vi "Change Camera Configuration.vi"(8 "error in (no error)":errorcluster, 10 "Camera Controls":T1={"VideoMode"=81, "Brightness"=150, "Sharpness"=50, "White Balance"=8000, "Saturation"=75, "Exposure"=5} {"VideoMode" items=["640 x 480 YUY 2 30.00 fps", "640 x 480 YUY 2 20.00 fps", "640 x 480 YUY 2 15.00 fps", "640 x 480 YUY 2 10.00 fps", "640 x 480 YUY 2 7.50 fps", "1280 x 720 YUY 2 10.00 fps", "1280 x 720 YUY 2 7.50 fps", "960 x 544 YUY 2 15.00 fps", "960 x 544 YUY 2 10.00 fps", "960 x 544 YUY 2 7.50 fps", "800 x 448 YUY 2 20.00 fps", "800 x 448 YUY 2 15.00 fps", "800 x 448 YUY 2 10.00 fps", "800 x 448 YUY 2 7.50 fps", "640 x 360 YUY 2 30.00 fps", "640 x 360 YUY 2 20.00 fps", "640 x 360 YUY 2 15.00 fps", "640 x 360 YUY 2 10.00 fps", "640 x 360 YUY 2 7.50 fps", "424 x 240 YUY 2 30.00 fps", "424 x 240 YUY 2 20.00 fps", "424 x 240 YUY 2 15.00 fps", "424 x 240 YUY 2 10.00 fps", "424 x 240 YUY 2 7.50 fps", "352 x 288 YUY 2 30.00 fps", "352 x 288 YUY 2 20.00 fps", "352 x 288 YUY 2 15.00 fps", "352 x 288 YUY 2 10.00 fps", "352 x 288 YUY 2 7.50 fps", "320 x 240 YUY 2 30.00 fps", "320 x 240 YUY 2 20.00 fps", "320 x 240 YUY 2 15.00 fps", "320 x 240 YUY 2 10.00 fps", "320 x 240 YUY 2 7.50 fps", "800 x 600 YUY 2 15.00 fps", "800 x 600 YUY 2 10.00 fps", "800 x 600 YUY 2 7.50 fps", "176 x 144 YUY 2 30.00 fps", "176 x 144 YUY 2 20.00 fps", "176 x 144 YUY 2 15.00 fps", "176 x 144 YUY 2 10.00 fps", "176 x 144 YUY 2 7.50 fps", "160 x 120 YUY 2 30.00 fps", "160 x 120 YUY 2 20.00 fps", "160 x 120 YUY 2 15.00 fps", "160 x 120 YUY 2 10.00 fps", "160 x 120 YUY 2 7.50 fps", "1280 x 800 YUY 2 10.00 fps", "640 x 480 JPEG 30.00 fps", "640 x 480 JPEG 20.00 fps", "640 x 480 JPEG 15.00 fps", "640 x 480 JPEG 10.00 fps", "640 x 480 JPEG 7.50 fps", "1280 x 720 JPEG 30.00 fps", "1280 x 720 JPEG 20.00 fps", "1280 x 720 JPEG 15.00 fps", "1280 x 720 JPEG 10.00 fps", "1280 x 720 JPEG 7.50 fps", "960 x 544 JPEG 30.00 fps", "960 x 544 JPEG 20.00 fps", "960 x 544 JPEG 15.00 fps", "960 x 544 JPEG 10.00 fps", "960 x 544 JPEG 7.50 fps", "800 x 448 JPEG 30.00 fps", "800 x 448 JPEG 20.00 fps", "800 x 448 JPEG 15.00 fps", "800 x 448 JPEG 10.00 fps", "800 x 448 JPEG 7.50 fps", "640 x 360 JPEG 30.00 fps", "640 x 360 JPEG 20.00 fps", "640 x 360 JPEG 15.00 fps", "640 x 360 JPEG 10.00 fps", "640 x 360 JPEG 7.50 fps", "800 x 600 JPEG 30.00 fps", "800 x 600 JPEG 20.00 fps", "800 x 600 JPEG 15.00 fps", "800 x 600 JPEG 10.00 fps", "800 x 600 JPEG 7.50 fps", "416 x 240 JPEG 30.00 fps", "416 x 240 JPEG 20.00 fps", "416 x 240 JPEG 15.00 fps", "416 x 240 JPEG 10.00 fps", "416 x 240 JPEG 7.50 fps", "352 x 288 JPEG 30.00 fps", "352 x 288 JPEG 20.00 fps", "352 x 288 JPEG 15.00 fps", "352 x 288 JPEG 10.00 fps", "352 x 288 JPEG 7.50 fps", "176 x 144 JPEG 30.00 fps", "176 x 144 JPEG 20.00 fps", "176 x 144 JPEG 15.00 fps", "176 x 144 JPEG 10.00 fps", "176 x 144 JPEG 7.50 fps", "320 x 240 JPEG 30.00 fps", "320 x 240 JPEG 20.00 fps", "320 x 240 JPEG 15.00 fps", "320 x 240 JPEG 10.00 fps", "320 x 240 JPEG 7.50 fps", "160 x 120 JPEG 30.00 fps", "160 x 120 JPEG 20.00 fps", "160 x 120 JPEG 15.00 fps", "160 x 120 JPEG 10.00 fps", "160 x 120 JPEG 7.50 fps"]}, 11 "Refnum In":T3={"Session"="", "Camera Settings"={"VideoMode"=81, "Brightness"=0, "Sharpness"=0, "White Balance"=0, "Saturation"=0, "Exposure"=0}} {"Camera Settings"."VideoMode" items=["640 x 480 YUY 2 30.00 fps", "640 x 480 YUY 2 20.00 fps", "640 x 480 YUY 2 15.00 fps", "640 x 480 YUY 2 10.00 fps", "640 x 480 YUY 2 7.50 fps", "1280 x 720 YUY 2 10.00 fps", "1280 x 720 YUY 2 7.50 fps", "960 x 544 YUY 2 15.00 fps", "960 x 544 YUY 2 10.00 fps", "960 x 544 YUY 2 7.50 fps", "800 x 448 YUY 2 20.00 fps", "800 x 448 YUY 2 15.00 fps", "800 x 448 YUY 2 10.00 fps", "800 x 448 YUY 2 7.50 fps", "640 x 360 YUY 2 30.00 fps", "640 x 360 YUY 2 20.00 fps", "640 x 360 YUY 2 15.00 fps", "640 x 360 YUY 2 10.00 fps", "640 x 360 YUY 2 7.50 fps", "424 x 240 YUY 2 30.00 fps", "424 x 240 YUY 2 20.00 fps", "424 x 240 YUY 2 15.00 fps", "424 x 240 YUY 2 10.00 fps", "424 x 240 YUY 2 7.50 fps", "352 x 288 YUY 2 30.00 fps", "352 x 288 YUY 2 20.00 fps", "352 x 288 YUY 2 15.00 fps", "352 x 288 YUY 2 10.00 fps", "352 x 288 YUY 2 7.50 fps", "320 x 240 YUY 2 30.00 fps", "320 x 240 YUY 2 20.00 fps", "320 x 240 YUY 2 15.00 fps", "320 x 240 YUY 2 10.00 fps", "320 x 240 YUY 2 7.50 fps", "800 x 600 YUY 2 15.00 fps", "800 x 600 YUY 2 10.00 fps", "800 x 600 YUY 2 7.50 fps", "176 x 144 YUY 2 30.00 fps", "176 x 144 YUY 2 20.00 fps", "176 x 144 YUY 2 15.00 fps", "176 x 144 YUY 2 10.00 fps", "176 x 144 YUY 2 7.50 fps", "160 x 120 YUY 2 30.00 fps", "160 x 120 YUY 2 20.00 fps", "160 x 120 YUY 2 15.00 fps", "160 x 120 YUY 2 10.00 fps", "160 x 120 YUY 2 7.50 fps", "1280 x 800 YUY 2 10.00 fps", "640 x 480 JPEG 30.00 fps", "640 x 480 JPEG 20.00 fps", "640 x 480 JPEG 15.00 fps", "640 x 480 JPEG 10.00 fps", "640 x 480 JPEG 7.50 fps", "1280 x 720 JPEG 30.00 fps", "1280 x 720 JPEG 20.00 fps", "1280 x 720 JPEG 15.00 fps", "1280 x 720 JPEG 10.00 fps", "1280 x 720 JPEG 7.50 fps", "960 x 544 JPEG 30.00 fps", "960 x 544 JPEG 20.00 fps", "960 x 544 JPEG 15.00 fps", "960 x 544 JPEG 10.00 fps", "960 x 544 JPEG 7.50 fps", "800 x 448 JPEG 30.00 fps", "800 x 448 JPEG 20.00 fps", "800 x 448 JPEG 15.00 fps", "800 x 448 JPEG 10.00 fps", "800 x 448 JPEG 7.50 fps", "640 x 360 JPEG 30.00 fps", "640 x 360 JPEG 20.00 fps", "640 x 360 JPEG 15.00 fps", "640 x 360 JPEG 10.00 fps", "640 x 360 JPEG 7.50 fps", "800 x 600 JPEG 30.00 fps", "800 x 600 JPEG 20.00 fps", "800 x 600 JPEG 15.00 fps", "800 x 600 JPEG 10.00 fps", "800 x 600 JPEG 7.50 fps", "416 x 240 JPEG 30.00 fps", "416 x 240 JPEG 20.00 fps", "416 x 240 JPEG 15.00 fps", "416 x 240 JPEG 10.00 fps", "416 x 240 JPEG 7.50 fps", "352 x 288 JPEG 30.00 fps", "352 x 288 JPEG 20.00 fps", "352 x 288 JPEG 15.00 fps", "352 x 288 JPEG 10.00 fps", "352 x 288 JPEG 7.50 fps", "176 x 144 JPEG 30.00 fps", "176 x 144 JPEG 20.00 fps", "176 x 144 JPEG 15.00 fps", "176 x 144 JPEG 10.00 fps", "176 x 144 JPEG 7.50 fps", "320 x 240 JPEG 30.00 fps", "320 x 240 JPEG 20.00 fps", "320 x 240 JPEG 15.00 fps", "320 x 240 JPEG 10.00 fps", "320 x 240 JPEG 7.50 fps", "160 x 120 JPEG 30.00 fps", "160 x 120 JPEG 20.00 fps", "160 x 120 JPEG 15.00 fps", "160 x 120 JPEG 10.00 fps", "160 x 120 JPEG 7.50 fps"]}) -> (0 "error out":errorcluster, 2 "Camera Controls Out":T1={"VideoMode"=81, "Brightness"=150, "Sharpness"=50, "White Balance"=8000, "Saturation"=75, "Exposure"=5} {"VideoMode" items=["640 x 480 YUY 2 30.00 fps", "640 x 480 YUY 2 20.00 fps", "640 x 480 YUY 2 15.00 fps", "640 x 480 YUY 2 10.00 fps", "640 x 480 YUY 2 7.50 fps", "1280 x 720 YUY 2 10.00 fps", "1280 x 720 YUY 2 7.50 fps", "960 x 544 YUY 2 15.00 fps", "960 x 544 YUY 2 10.00 fps", "960 x 544 YUY 2 7.50 fps", "800 x 448 YUY 2 20.00 fps", "800 x 448 YUY 2 15.00 fps", "800 x 448 YUY 2 10.00 fps", "800 x 448 YUY 2 7.50 fps", "640 x 360 YUY 2 30.00 fps", "640 x 360 YUY 2 20.00 fps", "640 x 360 YUY 2 15.00 fps", "640 x 360 YUY 2 10.00 fps", "640 x 360 YUY 2 7.50 fps", "424 x 240 YUY 2 30.00 fps", "424 x 240 YUY 2 20.00 fps", "424 x 240 YUY 2 15.00 fps", "424 x 240 YUY 2 10.00 fps", "424 x 240 YUY 2 7.50 fps", "352 x 288 YUY 2 30.00 fps", "352 x 288 YUY 2 20.00 fps", "352 x 288 YUY 2 15.00 fps", "352 x 288 YUY 2 10.00 fps", "352 x 288 YUY 2 7.50 fps", "320 x 240 YUY 2 30.00 fps", "320 x 240 YUY 2 20.00 fps", "320 x 240 YUY 2 15.00 fps", "320 x 240 YUY 2 10.00 fps", "320 x 240 YUY 2 7.50 fps", "800 x 600 YUY 2 15.00 fps", "800 x 600 YUY 2 10.00 fps", "800 x 600 YUY 2 7.50 fps", "176 x 144 YUY 2 30.00 fps", "176 x 144 YUY 2 20.00 fps", "176 x 144 YUY 2 15.00 fps", "176 x 144 YUY 2 10.00 fps", "176 x 144 YUY 2 7.50 fps", "160 x 120 YUY 2 30.00 fps", "160 x 120 YUY 2 20.00 fps", "160 x 120 YUY 2 15.00 fps", "160 x 120 YUY 2 10.00 fps", "160 x 120 YUY 2 7.50 fps", "1280 x 800 YUY 2 10.00 fps", "640 x 480 JPEG 30.00 fps", "640 x 480 JPEG 20.00 fps", "640 x 480 JPEG 15.00 fps", "640 x 480 JPEG 10.00 fps", "640 x 480 JPEG 7.50 fps", "1280 x 720 JPEG 30.00 fps", "1280 x 720 JPEG 20.00 fps", "1280 x 720 JPEG 15.00 fps", "1280 x 720 JPEG 10.00 fps", "1280 x 720 JPEG 7.50 fps", "960 x 544 JPEG 30.00 fps", "960 x 544 JPEG 20.00 fps", "960 x 544 JPEG 15.00 fps", "960 x 544 JPEG 10.00 fps", "960 x 544 JPEG 7.50 fps", "800 x 448 JPEG 30.00 fps", "800 x 448 JPEG 20.00 fps", "800 x 448 JPEG 15.00 fps", "800 x 448 JPEG 10.00 fps", "800 x 448 JPEG 7.50 fps", "640 x 360 JPEG 30.00 fps", "640 x 360 JPEG 20.00 fps", "640 x 360 JPEG 15.00 fps", "640 x 360 JPEG 10.00 fps", "640 x 360 JPEG 7.50 fps", "800 x 600 JPEG 30.00 fps", "800 x 600 JPEG 20.00 fps", "800 x 600 JPEG 15.00 fps", "800 x 600 JPEG 10.00 fps", "800 x 600 JPEG 7.50 fps", "416 x 240 JPEG 30.00 fps", "416 x 240 JPEG 20.00 fps", "416 x 240 JPEG 15.00 fps", "416 x 240 JPEG 10.00 fps", "416 x 240 JPEG 7.50 fps", "352 x 288 JPEG 30.00 fps", "352 x 288 JPEG 20.00 fps", "352 x 288 JPEG 15.00 fps", "352 x 288 JPEG 10.00 fps", "352 x 288 JPEG 7.50 fps", "176 x 144 JPEG 30.00 fps", "176 x 144 JPEG 20.00 fps", "176 x 144 JPEG 15.00 fps", "176 x 144 JPEG 10.00 fps", "176 x 144 JPEG 7.50 fps", "320 x 240 JPEG 30.00 fps", "320 x 240 JPEG 20.00 fps", "320 x 240 JPEG 15.00 fps", "320 x 240 JPEG 10.00 fps", "320 x 240 JPEG 7.50 fps", "160 x 120 JPEG 30.00 fps", "160 x 120 JPEG 20.00 fps", "160 x 120 JPEG 15.00 fps", "160 x 120 JPEG 10.00 fps", "160 x 120 JPEG 7.50 fps"]}, 3 "Refnum Out":T3={"Session"="", "Camera Settings"={"VideoMode"=81, "Brightness"=0, "Sharpness"=0, "White Balance"=0, "Saturation"=0, "Exposure"=0}} {"Camera Settings"."VideoMode" items=["640 x 480 YUY 2 30.00 fps", "640 x 480 YUY 2 20.00 fps", "640 x 480 YUY 2 15.00 fps", "640 x 480 YUY 2 10.00 fps", "640 x 480 YUY 2 7.50 fps", "1280 x 720 YUY 2 10.00 fps", "1280 x 720 YUY 2 7.50 fps", "960 x 544 YUY 2 15.00 fps", "960 x 544 YUY 2 10.00 fps", "960 x 544 YUY 2 7.50 fps", "800 x 448 YUY 2 20.00 fps", "800 x 448 YUY 2 15.00 fps", "800 x 448 YUY 2 10.00 fps", "800 x 448 YUY 2 7.50 fps", "640 x 360 YUY 2 30.00 fps", "640 x 360 YUY 2 20.00 fps", "640 x 360 YUY 2 15.00 fps", "640 x 360 YUY 2 10.00 fps", "640 x 360 YUY 2 7.50 fps", "424 x 240 YUY 2 30.00 fps", "424 x 240 YUY 2 20.00 fps", "424 x 240 YUY 2 15.00 fps", "424 x 240 YUY 2 10.00 fps", "424 x 240 YUY 2 7.50 fps", "352 x 288 YUY 2 30.00 fps", "352 x 288 YUY 2 20.00 fps", "352 x 288 YUY 2 15.00 fps", "352 x 288 YUY 2 10.00 fps", "352 x 288 YUY 2 7.50 fps", "320 x 240 YUY 2 30.00 fps", "320 x 240 YUY 2 20.00 fps", "320 x 240 YUY 2 15.00 fps", "320 x 240 YUY 2 10.00 fps", "320 x 240 YUY 2 7.50 fps", "800 x 600 YUY 2 15.00 fps", "800 x 600 YUY 2 10.00 fps", "800 x 600 YUY 2 7.50 fps", "176 x 144 YUY 2 30.00 fps", "176 x 144 YUY 2 20.00 fps", "176 x 144 YUY 2 15.00 fps", "176 x 144 YUY 2 10.00 fps", "176 x 144 YUY 2 7.50 fps", "160 x 120 YUY 2 30.00 fps", "160 x 120 YUY 2 20.00 fps", "160 x 120 YUY 2 15.00 fps", "160 x 120 YUY 2 10.00 fps", "160 x 120 YUY 2 7.50 fps", "1280 x 800 YUY 2 10.00 fps", "640 x 480 JPEG 30.00 fps", "640 x 480 JPEG 20.00 fps", "640 x 480 JPEG 15.00 fps", "640 x 480 JPEG 10.00 fps", "640 x 480 JPEG 7.50 fps", "1280 x 720 JPEG 30.00 fps", "1280 x 720 JPEG 20.00 fps", "1280 x 720 JPEG 15.00 fps", "1280 x 720 JPEG 10.00 fps", "1280 x 720 JPEG 7.50 fps", "960 x 544 JPEG 30.00 fps", "960 x 544 JPEG 20.00 fps", "960 x 544 JPEG 15.00 fps", "960 x 544 JPEG 10.00 fps", "960 x 544 JPEG 7.50 fps", "800 x 448 JPEG 30.00 fps", "800 x 448 JPEG 20.00 fps", "800 x 448 JPEG 15.00 fps", "800 x 448 JPEG 10.00 fps", "800 x 448 JPEG 7.50 fps", "640 x 360 JPEG 30.00 fps", "640 x 360 JPEG 20.00 fps", "640 x 360 JPEG 15.00 fps", "640 x 360 JPEG 10.00 fps", "640 x 360 JPEG 7.50 fps", "800 x 600 JPEG 30.00 fps", "800 x 600 JPEG 20.00 fps", "800 x 600 JPEG 15.00 fps", "800 x 600 JPEG 10.00 fps", "800 x 600 JPEG 7.50 fps", "416 x 240 JPEG 30.00 fps", "416 x 240 JPEG 20.00 fps", "416 x 240 JPEG 15.00 fps", "416 x 240 JPEG 10.00 fps", "416 x 240 JPEG 7.50 fps", "352 x 288 JPEG 30.00 fps", "352 x 288 JPEG 20.00 fps", "352 x 288 JPEG 15.00 fps", "352 x 288 JPEG 10.00 fps", "352 x 288 JPEG 7.50 fps", "176 x 144 JPEG 30.00 fps", "176 x 144 JPEG 20.00 fps", "176 x 144 JPEG 15.00 fps", "176 x 144 JPEG 10.00 fps", "176 x 144 JPEG 7.50 fps", "320 x 240 JPEG 30.00 fps", "320 x 240 JPEG 20.00 fps", "320 x 240 JPEG 15.00 fps", "320 x 240 JPEG 10.00 fps", "320 x 240 JPEG 7.50 fps", "160 x 120 JPEG 30.00 fps", "160 x 120 JPEG 20.00 fps", "160 x 120 JPEG 15.00 fps", "160 x 120 JPEG 10.00 fps", "160 x 120 JPEG 7.50 fps"]})   [LabVIEW 2015]
uses:
  Camera Data.ctl
  <vilib>/userdefined/High Color/IMAQdx.ctl
  Camera Settings.ctl
  Support Vision Code/38 Video Mode.ctl
  <resource>/objmgr/imaqdx.rc
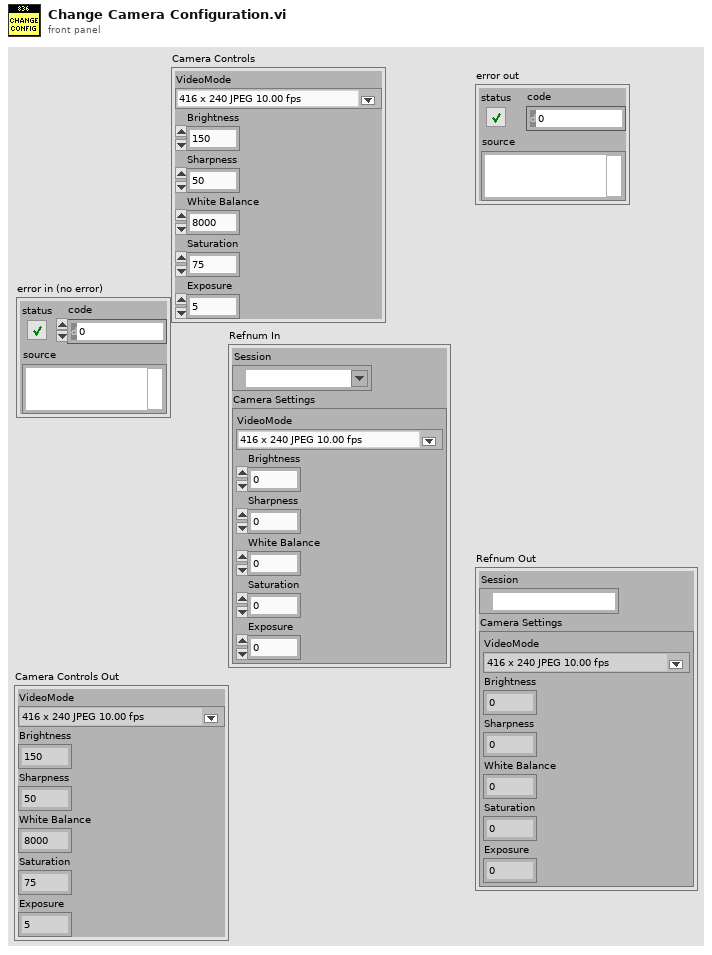
[diagram p1: front panel]
types:
  T1 = typedef "Camera Settings.ctl" = cluster{"VideoMode":T2, "Brightness":i32, "Sharpness":i32, "White Balance":i32, "Saturation":i32, "Exposure":i32}
  T2 = typedef "38 Video Mode.ctl" = u32
  T3 = typedef "Camera Data.ctl" = cluster{"Session":T4, "Camera Settings":T1}
  T4 = typedef "IMAQdx.ctl" = refnum<k21>
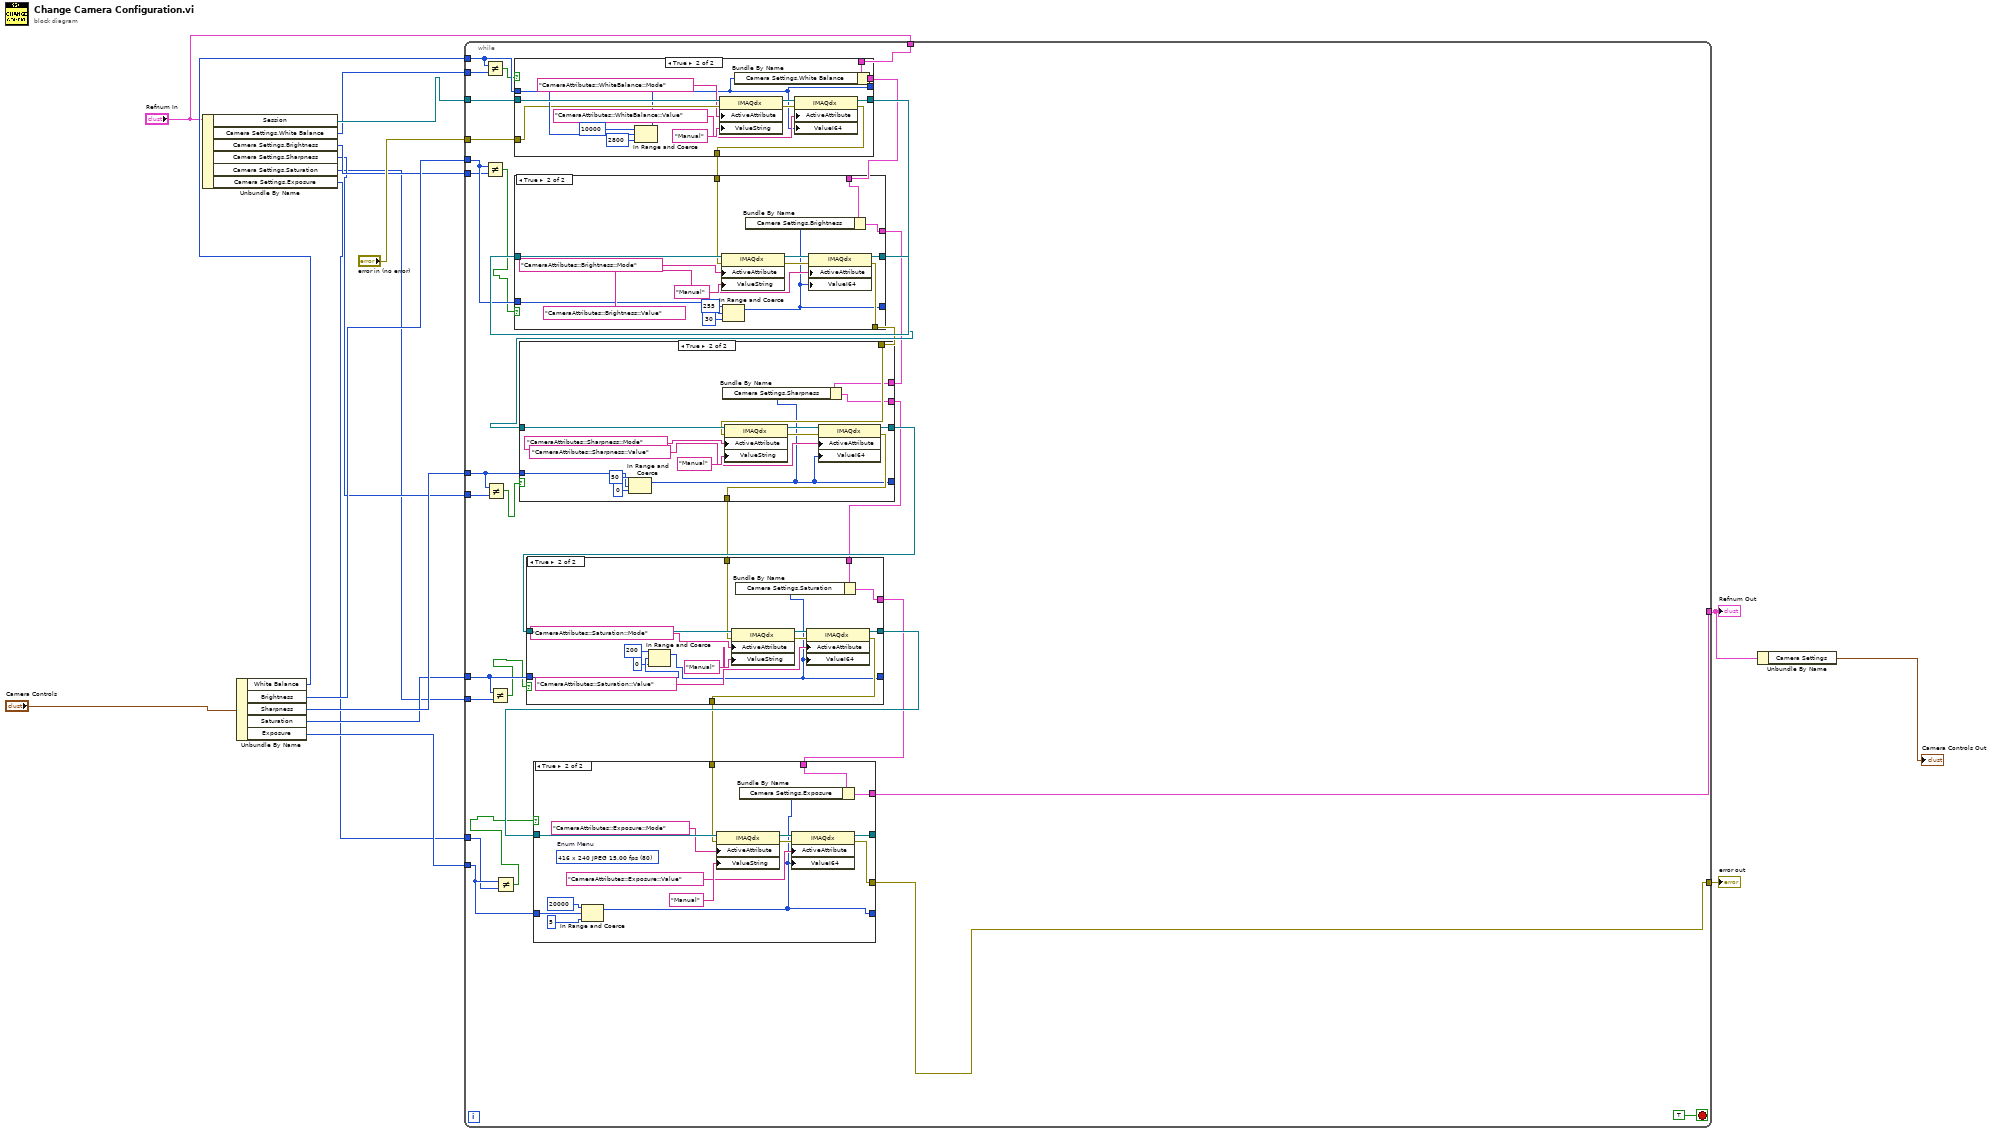
[diagram p0: block diagram]
diagram:
  n1 = Unbundle By Name("Refnum In") -> ("Session"=w10:T4, "Camera Settings.White Balance"=w9:i32, "Camera Settings.Brightness"=w8:i32, "Camera Settings.Sharpness"=w7:i32, "Camera Settings.Saturation"=w6:i32, "Camera Settings.Exposure"=w5:i32)
  n2 = Unbundle By Name("Camera Controls") -> ("White Balance"=w15:i32, "Brightness"=w14:i32, "Sharpness"=w13:i32, "Saturation"=w12:i32, "Exposure"=w11:i32)
  n3 = while {
    tunnel: w15 -> [w36]
    tunnel: w10 -> [w50]
    tunnel: w14 -> [w37]
    tunnel: w13 -> [w47]
    tunnel: w12 -> [w35]
    tunnel: w11 -> [w34]
    tunnel: [w38] -> w17
    tunnel: "error in (no error)" -> [w40]
    tunnel: w9 -> [w33]
    tunnel: w8 -> [w32]
    tunnel: w7 -> [w31]
    tunnel: w6 -> [w30]
    tunnel: w5 -> [w29]
    tunnel: "Refnum In" -> [w28]
    tunnel: [w23] -> w2
    stop <- TRUE stop-if-true
    n4 = Not Equal?(x=w36, y=w33) -> (x != y?=w18:bool)
    n5 = Not Equal?(x=w37, y=w32) -> (x != y?=w19:bool)
    n6 = Not Equal?(x=w47, y=w31) -> (x != y?=w20:bool)
    n7 = Not Equal?(x=w35, y=w30) -> (x != y?=w21:bool)
    n8 = Not Equal?(x=w34, y=w29) -> (x != y?=w22:bool)
    n9 = case shown="True" w18 {
      tunnel: w50 -> [w130 w144]
      tunnel: w36 -> [w128 w139]
      tunnel: [w130 w142] -> w49
      tunnel: [w129 w138] -> w39
      tunnel: w40 -> [w129 w136]
      tunnel: [w128 w132] -> _
      tunnel: w28 -> [w127 w133]
      tunnel: [w127 w131] -> w27
      frame False {
      }
      frame True {
        n10 = In Range and Coerce(upper limit=i64 10000, x=w139, lower limit=i64 2800) -> (coerced(x)=w132:i64)  [unwired: 1 out]
        n11 = property class="IMAQdx"(reference=w144, error in=w136, "ActiveAttribute"="CameraAttributes::WhiteBalance::Mode", "ValueString"="Manual") -> (reference out=w145:T4, error out=w137:errorcluster)
        n12 = Bundle By Name(cluster=w133, "Camera Settings.White Balance"=w132) -> (w131:T3)
        n13 = property class="IMAQdx"(reference=w145, error in=w137, "ActiveAttribute"="CameraAttributes::WhiteBalance::Value", "ValueI64"=w132) -> (reference out=w142:T4, error out=w138:errorcluster)
      }
    }
    n14 = case shown="True" w19 {
      tunnel: w49 -> [w111 w125]
      tunnel: [w111 w123] -> w48
      tunnel: w37 -> [w109 w119]
      tunnel: [w110 w118] -> w41
      tunnel: w39 -> [w110 w116]
      tunnel: [w109 w113] -> _
      tunnel: w27 -> [w108 w114]
      tunnel: [w108 w112] -> w26
      frame False {
      }
      frame True {
        n15 = property class="IMAQdx"(reference=w125, error in=w116, "ActiveAttribute"="CameraAttributes::Brightness::Mode", "ValueString"="Manual") -> (reference out=w126:T4, error out=w117:errorcluster)
        n16 = In Range and Coerce(upper limit=i64 255, x=w119, lower limit=i64 30) -> (coerced(x)=w113:i64)  [unwired: 1 out]
        n17 = Bundle By Name(cluster=w114, "Camera Settings.Brightness"=w113) -> (w112:T3)
        n18 = property class="IMAQdx"(reference=w126, error in=w117, "ActiveAttribute"="CameraAttributes::Brightness::Value", "ValueI64"=w113) -> (reference out=w123:T4, error out=w118:errorcluster)
      }
    }
    n19 = case shown="True" w20 {
      tunnel: w48 -> [w92 w106]
      tunnel: [w92 w104] -> w46
      tunnel: w47 -> [w90 w100]
      tunnel: [w91 w99] -> w42
      tunnel: w41 -> [w91 w97]
      tunnel: [w90 w93] -> _
      tunnel: w26 -> [w89 w95]
      tunnel: [w89 w94] -> w25
      frame False {
      }
      frame True {
        n20 = In Range and Coerce(upper limit=i64 50, x=w100, lower limit=i64 0) -> (coerced(x)=w93:i64)  [unwired: 1 out]
        n21 = Bundle By Name(cluster=w95, "Camera Settings.Sharpness"=w93) -> (w94:T3)
        n22 = property class="IMAQdx"(reference=w106, error in=w97, "ActiveAttribute"="CameraAttributes::Sharpness::Mode", "ValueString"="Manual") -> (reference out=w107:T4, error out=w98:errorcluster)
        n23 = property class="IMAQdx"(reference=w107, error in=w98, "ActiveAttribute"="CameraAttributes::Sharpness::Value", "ValueI64"=w93) -> (reference out=w104:T4, error out=w99:errorcluster)
      }
    }
    n24 = case shown="True" w21 {
      tunnel: w46 -> [w73 w87]
      tunnel: [w73 w85] -> w45
      tunnel: w35 -> [w71 w83]
      tunnel: [w72 w80] -> w43
      tunnel: w42 -> [w72 w78]
      tunnel: [w71 w75] -> _
      tunnel: w25 -> [w70 w76]
      tunnel: [w70 w74] -> w24
      frame False {
      }
      frame True {
        n25 = In Range and Coerce(upper limit=i64 200, x=w83, lower limit=i64 0) -> (coerced(x)=w75:i64)  [unwired: 1 out]
        n26 = property class="IMAQdx"(reference=w87, error in=w78, "ActiveAttribute"="CameraAttributes::Saturation::Mode", "ValueString"="Manual") -> (reference out=w88:T4, error out=w79:errorcluster)
        n27 = Bundle By Name(cluster=w76, "Camera Settings.Saturation"=w75) -> (w74:T3)
        n28 = property class="IMAQdx"(reference=w88, error in=w79, "ActiveAttribute"="CameraAttributes::Saturation::Value", "ValueI64"=w75) -> (reference out=w85:T4, error out=w80:errorcluster)
      }
    }
    n29 = case shown="True" w22 {
      tunnel: w45 -> [w54 w68]
      tunnel: [w54 w66] -> _
      tunnel: w34 -> [w52 w64]
      tunnel: [w53 w61] -> w38
      tunnel: w43 -> [w53 w59]
      tunnel: [w52 w55] -> _
      tunnel: w24 -> [w51 w57]
      tunnel: [w51 w56] -> w23
      frame False {
      }
      frame True {
        (unwired) T2 80 items=["640 x 480 YUY 2 30.00 fps", "640 x 480 YUY 2 20.00 fps", "640 x 480 YUY 2 15.00 fps", "640 x 480 YUY 2 10.00 fps", "640 x 480 YUY 2 7.50 fps", "1280 x 720 YUY 2 10.00 fps", "1280 x 720 YUY 2 7.50 fps", "960 x 544 YUY 2 15.00 fps", "960 x 544 YUY 2 10.00 fps", "960 x 544 YUY 2 7.50 fps", "800 x 448 YUY 2 20.00 fps", "800 x 448 YUY 2 15.00 fps", "800 x 448 YUY 2 10.00 fps", "800 x 448 YUY 2 7.50 fps", "640 x 360 YUY 2 30.00 fps", "640 x 360 YUY 2 20.00 fps", "640 x 360 YUY 2 15.00 fps", "640 x 360 YUY 2 10.00 fps", "640 x 360 YUY 2 7.50 fps", "424 x 240 YUY 2 30.00 fps", "424 x 240 YUY 2 20.00 fps", "424 x 240 YUY 2 15.00 fps", "424 x 240 YUY 2 10.00 fps", "424 x 240 YUY 2 7.50 fps", "352 x 288 YUY 2 30.00 fps", "352 x 288 YUY 2 20.00 fps", "352 x 288 YUY 2 15.00 fps", "352 x 288 YUY 2 10.00 fps", "352 x 288 YUY 2 7.50 fps", "320 x 240 YUY 2 30.00 fps", "320 x 240 YUY 2 20.00 fps", "320 x 240 YUY 2 15.00 fps", "320 x 240 YUY 2 10.00 fps", "320 x 240 YUY 2 7.50 fps", "800 x 600 YUY 2 15.00 fps", "800 x 600 YUY 2 10.00 fps", "800 x 600 YUY 2 7.50 fps", "176 x 144 YUY 2 30.00 fps", "176 x 144 YUY 2 20.00 fps", "176 x 144 YUY 2 15.00 fps", "176 x 144 YUY 2 10.00 fps", "176 x 144 YUY 2 7.50 fps", "160 x 120 YUY 2 30.00 fps", "160 x 120 YUY 2 20.00 fps", "160 x 120 YUY 2 15.00 fps", "160 x 120 YUY 2 10.00 fps", "160 x 120 YUY 2 7.50 fps", "1280 x 800 YUY 2 10.00 fps", "640 x 480 JPEG 30.00 fps", "640 x 480 JPEG 20.00 fps", "640 x 480 JPEG 15.00 fps", "640 x 480 JPEG 10.00 fps", "640 x 480 JPEG 7.50 fps", "1280 x 720 JPEG 30.00 fps", "1280 x 720 JPEG 20.00 fps", "1280 x 720 JPEG 15.00 fps", "1280 x 720 JPEG 10.00 fps", "1280 x 720 JPEG 7.50 fps", "960 x 544 JPEG 30.00 fps", "960 x 544 JPEG 20.00 fps", "960 x 544 JPEG 15.00 fps", "960 x 544 JPEG 10.00 fps", "960 x 544 JPEG 7.50 fps", "800 x 448 JPEG 30.00 fps", "800 x 448 JPEG 20.00 fps", "800 x 448 JPEG 15.00 fps", "800 x 448 JPEG 10.00 fps", "800 x 448 JPEG 7.50 fps", "640 x 360 JPEG 30.00 fps", "640 x 360 JPEG 20.00 fps", "640 x 360 JPEG 15.00 fps", "640 x 360 JPEG 10.00 fps", "640 x 360 JPEG 7.50 fps", "800 x 600 JPEG 30.00 fps", "800 x 600 JPEG 20.00 fps", "800 x 600 JPEG 15.00 fps", "800 x 600 JPEG 10.00 fps", "800 x 600 JPEG 7.50 fps", "416 x 240 JPEG 30.00 fps", "416 x 240 JPEG 20.00 fps", "416 x 240 JPEG 15.00 fps", "416 x 240 JPEG 10.00 fps", "416 x 240 JPEG 7.50 fps", "352 x 288 JPEG 30.00 fps", "352 x 288 JPEG 20.00 fps", "352 x 288 JPEG 15.00 fps", "352 x 288 JPEG 10.00 fps", "352 x 288 JPEG 7.50 fps", "176 x 144 JPEG 30.00 fps", "176 x 144 JPEG 20.00 fps", "176 x 144 JPEG 15.00 fps", "176 x 144 JPEG 10.00 fps", "176 x 144 JPEG 7.50 fps", "320 x 240 JPEG 30.00 fps", "320 x 240 JPEG 20.00 fps", "320 x 240 JPEG 15.00 fps", "320 x 240 JPEG 10.00 fps", "320 x 240 JPEG 7.50 fps", "160 x 120 JPEG 30.00 fps", "160 x 120 JPEG 20.00 fps", "160 x 120 JPEG 15.00 fps", "160 x 120 JPEG 10.00 fps", "160 x 120 JPEG 7.50 fps"]  # Enum Menu
        n30 = In Range and Coerce(upper limit=i64 20000, x=w64, lower limit=i64 5) -> (coerced(x)=w55:i64)  [unwired: 1 out]
        n31 = property class="IMAQdx"(reference=w68, error in=w59, "ActiveAttribute"="CameraAttributes::Exposure::Mode", "ValueString"="Manual") -> (reference out=w69:T4, error out=w60:errorcluster)
        n32 = Bundle By Name(cluster=w57, "Camera Settings.Exposure"=w55) -> (w56:T3)
        n33 = property class="IMAQdx"(reference=w69, error in=w60, "ActiveAttribute"="CameraAttributes::Exposure::Value", "ValueI64"=w55) -> (reference out=w66:T4, error out=w61:errorcluster)
      }
    }
  }
  "error out" <- w17
  "Refnum Out" <- w2
  n34 = Unbundle By Name(w2) -> ("Camera Settings"=→"Camera Controls Out":T1)
